vi "在表格最后插入列.vi"(8 "错误输入（无错误）":errorcluster, 10 "内容":string[](array[string]), 11 "引用输入":refnum<vi>) -> (0 "错误输出":errorcluster, 3 "引用输出":refnum<vi>)   [LabVIEW 2014, in "表格.lvlib"]
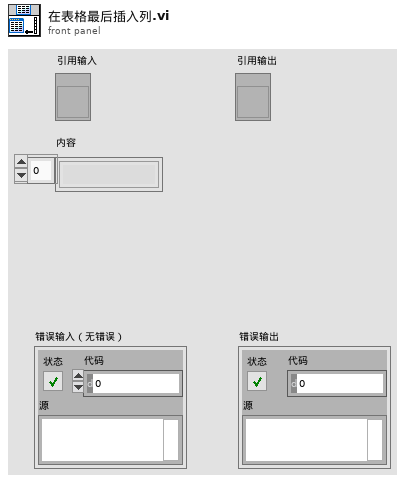
[diagram p1: front panel]
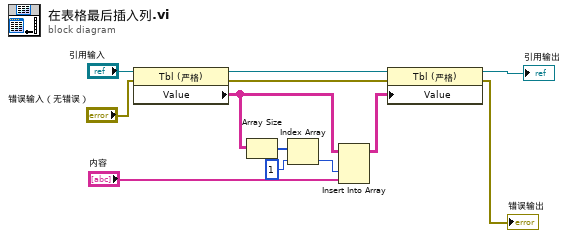
[diagram p0: block diagram]
diagram:
  n1 = property class="Tbl (严格)"(reference="引用输入", error in="错误输入（无错误）") -> (reference out=w12:refnum<vi>, error out=w11:errorcluster, "Value"=w4:string[][])
  n2 = Array Size(array=w4) -> (size(s)=w7:i32[])
  n3 = Index Array(array=w7, index=1 ("索引")) -> (element=w3:i32)
  n4 = Insert Into Array(array=w4, index (col)=w3, new element="内容") -> (w1:string[][])  [unwired: 1 in]
  n5 = property class="Tbl (严格)"(reference=w12, error in=w11, "Value"=w1) -> (reference out=→"引用输出":refnum<vi>, error out=→"错误输出":errorcluster)
